vi "second.vi"() -> ()   [LabVIEW 2019]
panel:
  in  "Slide":dbl(slide) scale=0.0..10.0
  out "Gauge":dbl(knob) scale=0.0..10.0
  out "Boolean":bool
  in  "button2":bool
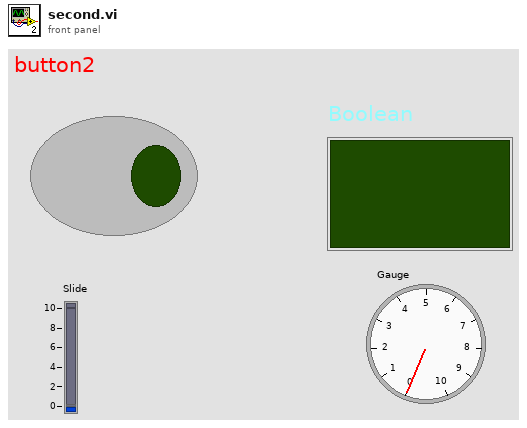
[diagram p1: front panel]
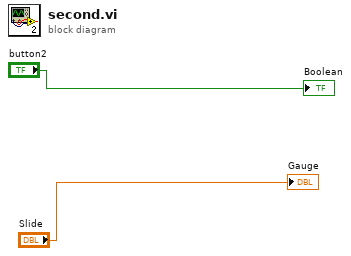
[diagram p0: block diagram]
diagram:
  "Boolean" <- "button2"
  "Gauge" <- "Slide"
